vi "Find VIs not in project.vi"() -> ()   [LabVIEW 2019]
uses:
  121e7d09-ebae-4b13-9a92-67fd7773fd38.vi
panel:
  out "Array":path[](array[path])
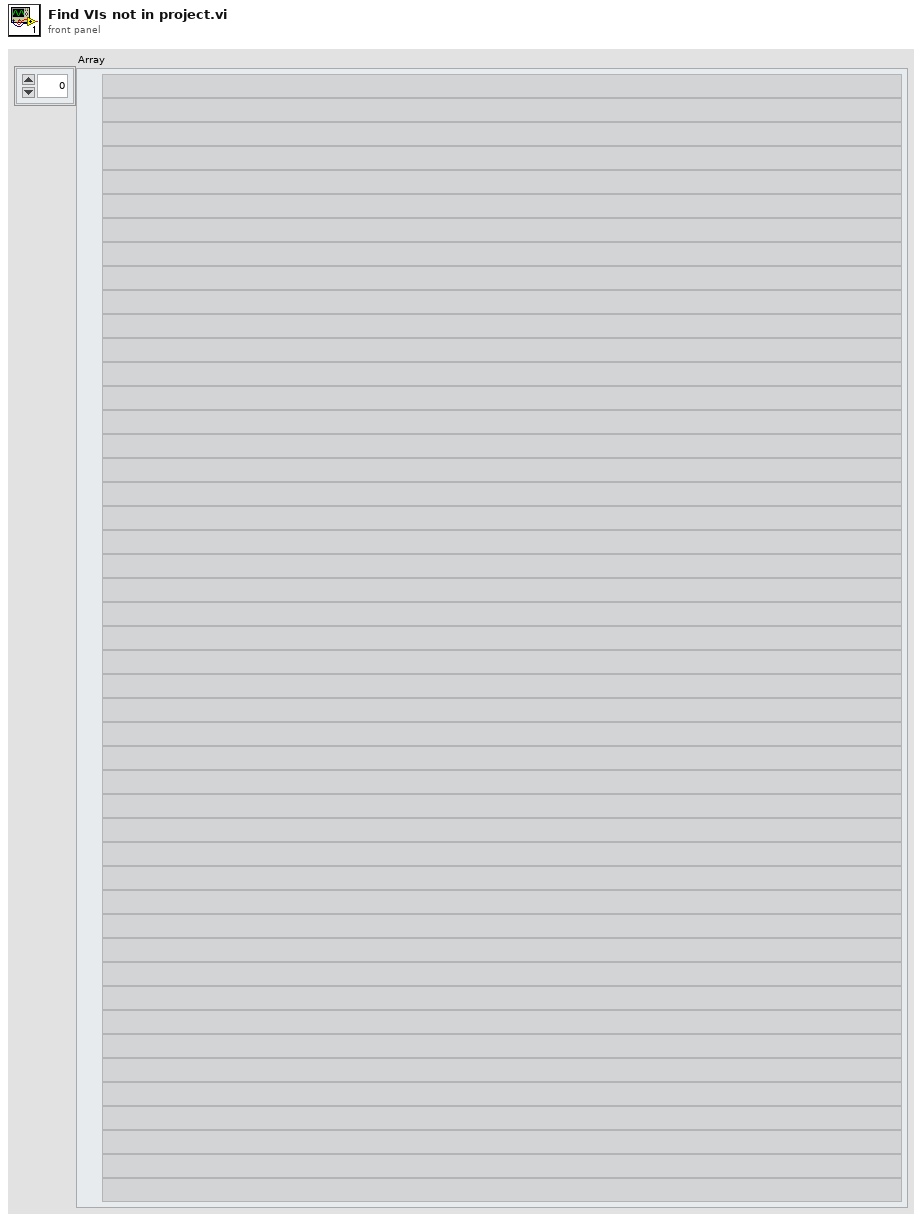
[diagram p1: front panel]
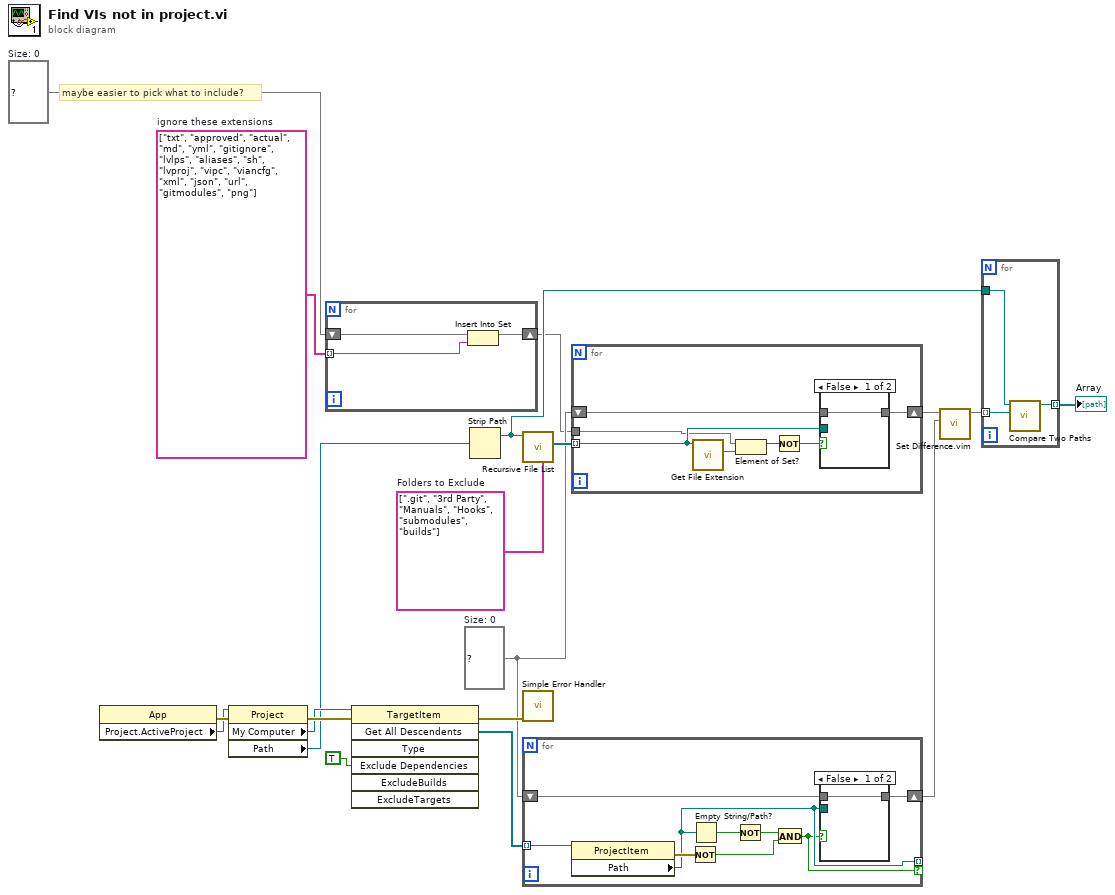
[diagram p0: block diagram]
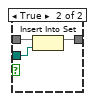
[diagram p2: hidden frame]
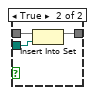
[diagram p3: hidden frame]
diagram:
  w2 = string[] ["txt", "approved", "actual", "md", "yml", "gitignore", "lvlps", "aliases", "sh", "lvproj", "vipc", "viancfg", "xml", "json", "url", "gitmodules", "png"]  # ignore these extensions
  w4 = set{string} {}  # Size: 0
  w5 = string[] [".git", "3rd Party", "Manuals", "Hooks", "submodules", "builds"]  # Folders to Exclude
  w11 = set{path} {}  # Size: 0
  # "maybe easier to pick what to include?"
  n1 = property class="App"() -> (error out=w19:errorcluster, "Project.ActiveProject"=w16:refnum<vi>)  [unwired: 2 in, 1 out]
  n2 = property class="Project"(reference=w16, error in=w19) -> (error out=w18:errorcluster, "My Computer"=w15:refnum<vi>, "Path"=w13:path)  [unwired: 1 out]
  n3 = for {
    shift-right: [w21] -> w3
    shift-left: w4 -> [w22]
    tunnel: w2 -> [w20] mode=indexing
    n4 = Insert Into Set(10:w20, 11:w22) -> (3:w21:set{string})  [unwired: 1 out]
  }
  n5 = invoke class="TargetItem" method="Get All Descendents"(reference=w15, error in=w18, "Exclude Dependencies"=TRUE ("ExcludeDependencies")) -> (error out=w17:errorcluster, "All Descendents"=w14:refnum<vi>[])  [unwired: 4 in, 5 out]
  n6 = Strip Path(path=w13) -> (stripped path=w7:path)  [unwired: 1 out]
  n7 = call <vilib>:"Recursive File List.vi"("Folders to Exclude"=w5, "Folder Path"=w7) -> ("All Files in Dir"=w12:path[])  [unwired: 5 in, 4 out]
  n8 = call <vilib>:"Simple Error Handler.vi"("error in (no error)"=w17) -> ()  [unwired: 4 in, 5 out]
  n9 = for {
    tunnel: w14 -> [w30] mode=indexing
    tunnel: [w24] -> _ mode=indexing if=w23
    shift-right: [w25] -> w9
    shift-left: w11 -> [w26]
    n10 = property class="ProjectItem"(reference=w30) -> (error out=w31:errorcluster, "Path"=w24:path)  [unwired: 1 in, 1 out]
    n11 = Not(x=w31) -> (.not. x?=w29:bool)
    n12 = Empty String/Path?(string/path=w24) -> (empty?=w27:bool)
    n13 = Not(x=w27) -> (.not. x?=w28:bool)
    n14 = And(x=w28, y=w29) -> (x .and. y?=w23:bool)
    n15 = case shown="False" w23 {
      tunnel: w26 -> [w32 w35]
      tunnel: [w32 w34] -> w25
      tunnel: w24 -> [_ w33]
      frame False {
      }
      frame True {
        n16 = Insert Into Set(10:w33, 11:w35) -> (3:w34:set{path})  [unwired: 1 out]
      }
    }
  }
  n17 = for {
    shift-right: [w41] -> w10
    shift-left: w11 -> [w42]
    tunnel: w12 -> [w40] mode=indexing
    tunnel: w3 -> [w39]
    n18 = call <vilib>:"Get File Extension.vi"("file"=w40) -> ("lowercase file extension"=w38:string)  [unwired: 6 in, 4 out]
    n19 = Element of Set?(10:w38, 11:w39) -> (3:w37:bool)
    n20 = Not(x=w37) -> (.not. x?=w36:bool)
    n21 = case shown="False" w36 {
      tunnel: w42 -> [w43 w46]
      tunnel: [w43 w45] -> w41
      tunnel: w40 -> [_ w44]
      frame False {
      }
      frame True {
        n22 = Insert Into Set(10:w44, 11:w46) -> (3:w45:set{path})  [unwired: 1 out]
      }
    }
  }
  n23 = call "Set Difference.vim"("set 2"=w9, "set 1"=w10) -> ("difference"=w8:set{path})  [unwired: 9 in]
  n24 = for {
    tunnel: w8 -> [w47] mode=indexing
    tunnel: w7 -> [w48]
    tunnel: [w49] -> w6 mode=indexing
    n25 = call <vilib>:"Compare Two Paths.vi"("Path 2"=w47, "Path 1"=w48) -> ("Relative Path from 1 to 2"=w49:path)  [unwired: 6 in, 3 out]
  }
  "Array" <- w6
